vi "Stop Core.vi"(10 "final error code":i32, 11 "PLC_Module in":refnum<class "PLC_Module.lvclass">) -> (3 "PLC_Module out":refnum<class "PLC_Module.lvclass">)   [LabVIEW 2025, in "PLC_Module.lvlib" / "PLC_Module.lvclass"]
doc: "<p>(<strong>Filename</strong>: <span class=\"dnl\">Actor Framework.lvlib:Actor.lvclass:Stop Core.vi</span>)</p>\n<p>Defines what the actor does before it stops. Use the <strong>final error code</strong> input to determine whether the actor shut down in response to an error.</p>\n<p>By default, this method passes the Stop message along to all <a href=\"nihelplauncher://docs/csh?context=lvcore_lvcomm_af_launch_nested_actor\">auto-stop nested actors</a>. A descendant class may override this method to define additional behavior, such as shutting down any processes the actor initiated in its override of the <a href=\"nihelplauncher://docs/csh?context=lvcore_lvcomm_af_actor_core\">Actor Core</a> method.</p>"
uses:
  PLC_Module.lvclass
  Msg.ctl
  PLC_Module.lvclass/PLC_Module.ctl
  <vilib>/ActorFramework/Actor/Actor.lvclass
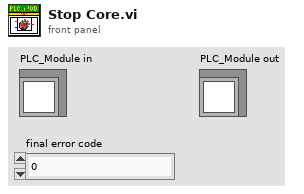
[diagram p1: front panel]
types:
  T1 = typedef "Msg.ctl" = string
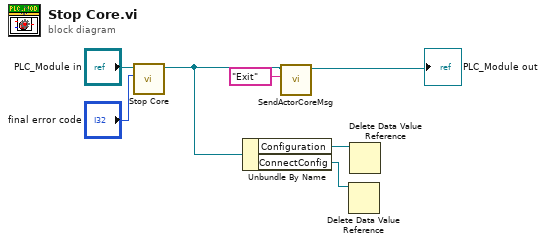
[diagram p0: block diagram]
diagram:
  n1 = call-parent "Stop Core.vi"("final error code"="final error code", "Actor in"="PLC_Module in") -> ("Actor out"=w3:refnum<class "PLC_Module.lvclass">)  [unwired: 9 in]
  n2 = Unbundle By Name(w3) -> ("Configuration"=w2:refnum<data-value>, "ConnectConfig"=w1:refnum<data-value>)
  n3 = call "SendActorCoreMsg.vi"("Msg"=T1 "Exit", "PLC_Module in"=w3) -> ("PLC_Module out"=→"PLC_Module out":refnum<class "PLC_Module.lvclass">)  [unwired: 8 in, 1 out]
  n4 = Delete Data Value Reference(data value reference=w1) -> ()  [unwired: 1 in, 2 out]
  n5 = Delete Data Value Reference(data value reference=w2) -> ()  [unwired: 1 in, 2 out]
